vi "LoadIniRegExtSession.vi"(8 "error in (no error)":errorcluster) -> (0 "error out":errorcluster, 3 "RegExt":T1)   [LabVIEW 2014]
uses:
  control/DEF-RegExt.ctl
  <vilib>/Utility/config.llb/NI_LVConfig.lvlib
  application.lvclass
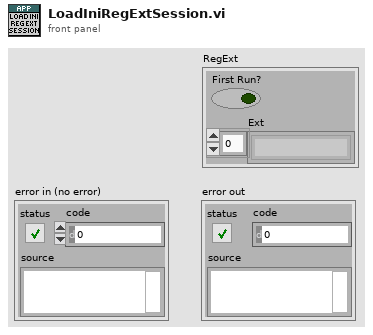
[diagram p1: front panel]
types:
  T1 = typedef "application.lvclass/DEF-RegExt.ctl" = cluster{"First Run?":bool, "Ext":string[]}
  T2 = typedef "NI_LVConfig.lvlib/Config Data RefNum.ctl" = refnum<k1>
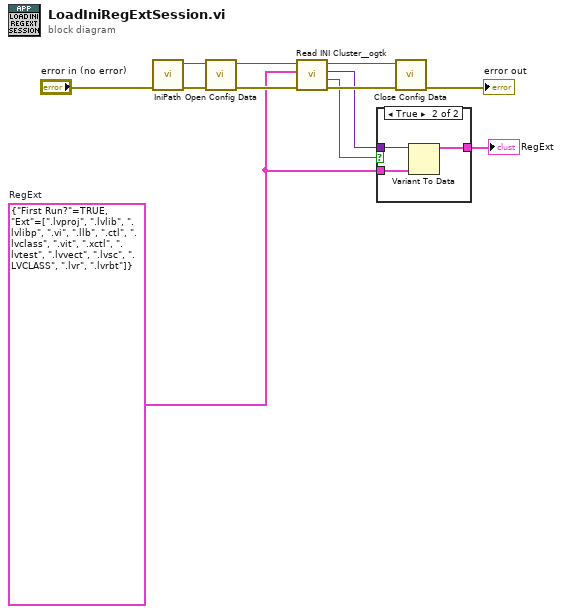
[diagram p0: block diagram]
diagram:
  w3 = T1 {"First Run?"=TRUE, "Ext"=[".lvproj", ".lvlib", ".lvlibp", ".vi", ".llb", ".ctl", ".lvclass", ".vit", ".xctl", ".lvtest", ".lvvect", ".lvsc", ".LVCLASS", ".lvr", ".lvrbt"]}  # RegExt
  n1 = call "IniPath.vi"() -> ("INI Path"=w11:path)  [unwired: 11 in]
  n2 = call <vilib>:"Open Config Data.vi"("error in (no error)"="error in (no error)", "configuration file path"=w11) -> ("error out"=w5:errorcluster, "refnum"=w6:T2)  [unwired: 7 in, 1 out]
  n3 = call <userlib>:"Read INI Cluster__ogtk.vi"("error in (no error)"=w5, "INI Fomatted Cluster Type"=w3, "refnum"=w6) -> ("error out"=w9:errorcluster, "all found?"=w1:bool, "INI Fomatted Cluster"=w4:variant, "dup refnum"=w8:T2)  [unwired: 4 in, 1 out]
  n4 = case shown="True" w1 {
    tunnel: w4 -> [_ w15]
    tunnel: w3 -> [w12 w14]
    tunnel: [w12 w13] -> w2
    frame False {
    }
    frame True {
      n5 = Variant To Data(type=w14, Variant=w15) -> (data=w13:T1)  [unwired: 1 in, 1 out]
    }
  }
  "RegExt" <- w2
  n6 = call <vilib>:"Close Config Data.vi"("error in (no error)"=w9, "refnum"=w8) -> ("error out"=→"error out":errorcluster)  [unwired: 8 in, 1 out]
